vi "Set Display String.vi"(8 "error in(no error)":errorcluster, 10 "display string (none)":string, 11 "VISA Resource Name":refnum<visa-resource-name>) -> (0 "error out":errorcluster, 3 "VISA resource name out":refnum<visa-resource-name>)   [LabVIEW 2020, in "3458A Virtual Digitizer.lvlib" / "3458A Basic Driver.lvlib"]
doc: "Sets display message."
uses:
  3458A Basic Driver.lvlib
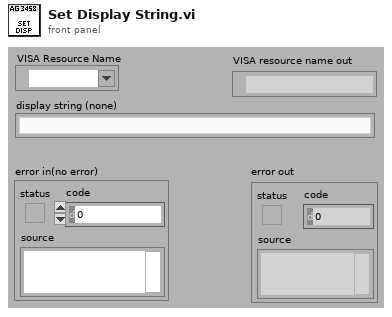
[diagram p1: front panel]
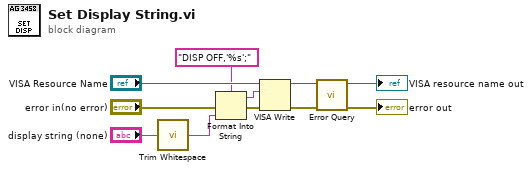
[diagram p0: block diagram]
diagram:
  n1 = call <vilib>:"Trim Whitespace.vi"("string"="display string (none)") -> ("trimmed string"=w5:string)  [unwired: 1 in]
  n2 = Format Into String(format string="DISP OFF,'%s';" ("write buffer"), error in="error in(no error)", w5) -> (resulting string=w8:string, error out=w10:errorcluster)  [unwired: 1 in]
  n3 = VISA Write(VISA resource name="VISA Resource Name", write buffer=w8, error in (no error)=w10) -> (VISA resource name out=w3:refnum<visa-resource-name>, error out=w4:errorcluster)  [unwired: 1 out]
  n4 = call "Error Query.vi"("error in (no error)"=w4, "VISA resource name"=w3) -> ("error out"=→"error out":errorcluster, "VISA resource name out"=→"VISA resource name out":refnum<visa-resource-name>)  [unwired: 6 in, 2 out]
